vi "Set_TestInformaton.vi"(8 "error in (no error)":errorcluster caption="错误输入（无错误）", 10 "TestInformaton":string[](array[string])=["EnabledBarcode", "Length", "Environment", "CustomerName", "OrderNumber", "FailRateMax", "Inspector", "Repeat", "MES", "CSV", "TXT", "XML", "TestFixtureNumber"], 11 "路径":path) -> (0 "error out":errorcluster caption="错误输出", 3 "路径 2":path)   [LabVIEW 2018]
uses:
  Global.vi
  <vilib>/Utility/config.llb/Write Key (String).vi
  <vilib>/Utility/config.llb/NI_LVConfig.lvlib
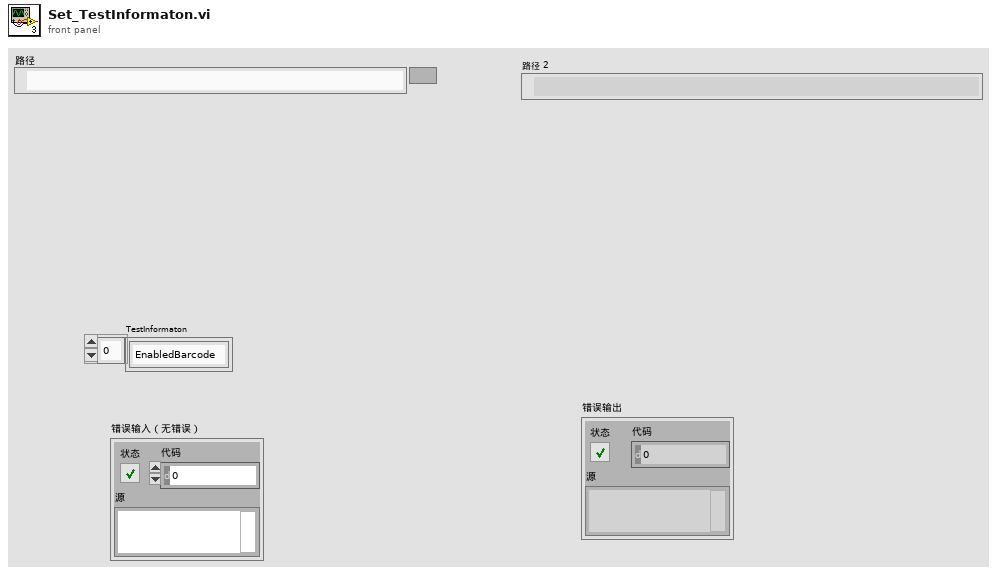
[diagram p1: front panel]
types:
  T1 = typedef "NI_LVConfig.lvlib/Config Data RefNum.ctl" = refnum<k1>
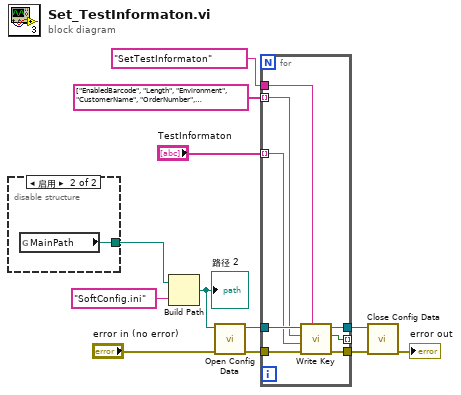
[diagram p0: block diagram]
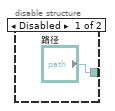
[diagram p2: hidden frame]
diagram:
  n1 = disable-structure shown="启用" {
    disable-tunnel: ["路径" w14] -> w7
    frame Disabled {
    }
    frame Enabled {
      n2 = global read "Global.vi" "MainPath"() -> (w14:path)
    }
  }
  n3 = Build Path(base path=w7, name or relative path="SoftConfig.ini" ("名称或相对路径")) -> (appended path=w5:path)
  "路径 2" <- w5
  n4 = call <vilib>:"Open Config Data.vi"("error in (no error)"="error in (no error)", "configuration file path"=w5) -> ("error out"=w4:errorcluster, "refnum"=w3:T1)  [unwired: 7 in, 1 out]
  n5 = for {
    tunnel: string[] ["EnabledBarcode", "Length", "Environment", "CustomerName", "OrderNumber", "FailRateMax", "Inspector", "Repeat", "MES", "CSV", "TXT", "XML", "TestFixtureNumber"] -> [w21] mode=indexing
    tunnel: w3 -> [w22]
    tunnel: [w20] -> _ mode=indexing
    tunnel: [w19] -> w8
    tunnel: "SetTestInformaton" ("section") -> [w18]
    tunnel: [w17] -> w10
    tunnel: w4 -> [w16]
    tunnel: "TestInformaton" -> [w15] mode=indexing
    n6 = call-poly <vilib>:"Write Key.vi"("section"=w18, "error in (no error)"=w16, "value"=w15, "key"=w21, "refnum"=w22) -> ("error out"=w17:errorcluster, "found?"=w20:bool, "refnum out"=w19:T1)  [unwired: 4 in]
  }
  n7 = call <vilib>:"Close Config Data.vi"("error in (no error)"=w10, "refnum"=w8) -> ("error out"=→"error out":errorcluster)  [unwired: 8 in, 1 out]
